vi "Perform Action.vi"(8 "error in (no error)":errorcluster, 10 "Input":variant, 11 "Virt PWM Fixed Freq Generator in":refnum<class "Virt DAQmx Fixed Freq PWM Generator.lvclass">) -> (0 "error out":errorcluster, 2 "Output":variant, 3 "Virt PWM Fixed Freq Generator out":refnum<class "Virt DAQmx Fixed Freq PWM Generator.lvclass">)   [LabVIEW 2023, in "Virt Instrs DIO.lvlib" / "Virt DAQmx Fixed Freq PWM Generator.lvclass"]
uses:
  Virt DAQmx Fixed Freq PWM Generator.lvclass
  Virt DAQmx Fixed Freq PWM Generator.lvclass/Virt DAQmx Fixed Freq PWM Generator.ctl
  Virt Instr Host/Virt Instr Local.lvclass
  Instrument/Instrument.lvclass
  Virt Instr Base/Virt Instr Base.lvclass
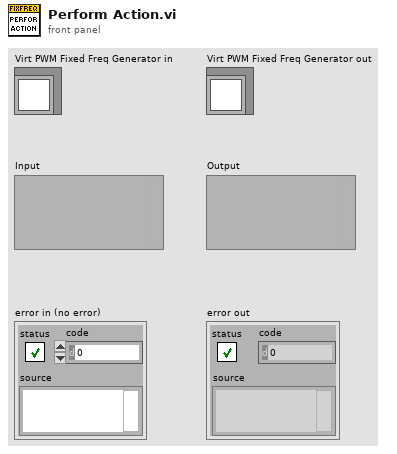
[diagram p1: front panel]
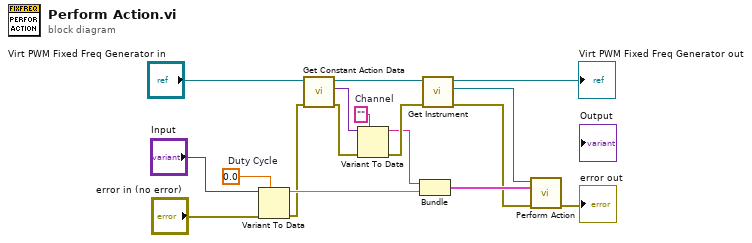
[diagram p0: block diagram]
diagram:
  w1 = 0.0  # Duty Cycle
  w13 = ""  # Channel
  n1 = Variant To Data(error in="error in (no error)", type=w1, Variant="Input") -> (data=w17:dbl, error out=w15:errorcluster)
  n2 = call "Get Constant Action Data.vi"("error in (no error)"=w15, "Virt Instr Base in"="Virt PWM Fixed Freq Generator in") -> ("error out"=w16:errorcluster, "Constant Action Data"=w10:variant, "Virt Instr Base out"=w11:refnum<class "Virt DAQmx Fixed Freq PWM Generator.lvclass">)  [unwired: 7 in]
  n3 = Variant To Data(error in=w16, type=w13, Variant=w10) -> (data=w12:string, error out=w14:errorcluster)
  n4 = Bundle("Channel"=w12, "Duty Cycle"=w17) -> (w9:cluster{"Channel":string, "Duty Cycle":dbl})  [unwired: 1 in]
  n5 = call "Get Instrument.vi"("error in (no error)"=w14, "Virt Instr Base in"=w11) -> ("error out"=w7:errorcluster, "HAL GOOP4.lvlib:Instrument"=w8:refnum<class "Instrument.lvclass">, "Virt Instr Base out"=→"Virt PWM Fixed Freq Generator out":refnum<class "Virt DAQmx Fixed Freq PWM Generator.lvclass">)  [unwired: 7 in]
  n6 = call "Perform Action.vi"("Error In"=w7, "Input"=w9, "reference in"=w8) -> ("Error Out"=→"error out":errorcluster)  [unwired: 6 in, 2 out]
